vi "LaserStatus.vi"() -> (0 "h1-transmission":dbl format="%.2f", 1 "rep-rate":dbl format="%.2f", 2 "hu-error-code":i32, 3 "laser-error-code":i32, 4 "h1-zero-transmission-offset":i32, 5 "HU-Temp-Ready?":bool, 6 "LD1-set-current":dbl format="%.2f", 7 "LaserOn?":bool)   [LabVIEW 2020]
uses:
  <vilib>/JDP Science/JSONtext/String Subset.vi
  <vilib>/JDP Science/JSONtext/Parsing/Parse Full Path or Item Name.vi
  <vilib>/JDP Science/JSONtext/Next JSON Value.vi
  <vilib>/JDP Science/JSONtext/support/Error Cluster From Code.vi
  <vilib>/JDP Science/JSONtext/Offset/Find Item Locations by Path.vi
  <vilib>/httpClient/LabVIEWHTTPClient.lvlib
  <vilib>/JDP Science/JSONtext/JSONtext.lvlib
panel:
  out "body":string
  out "headers":string
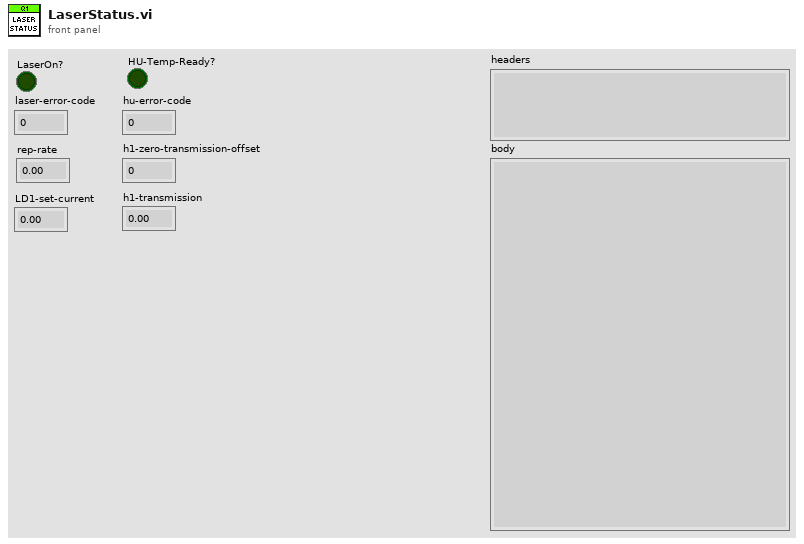
[diagram p1: front panel]
types:
  T1 = typedef "LabVIEWHTTPClient.lvlib/ClientHandle.ctl" = refnum<k1>
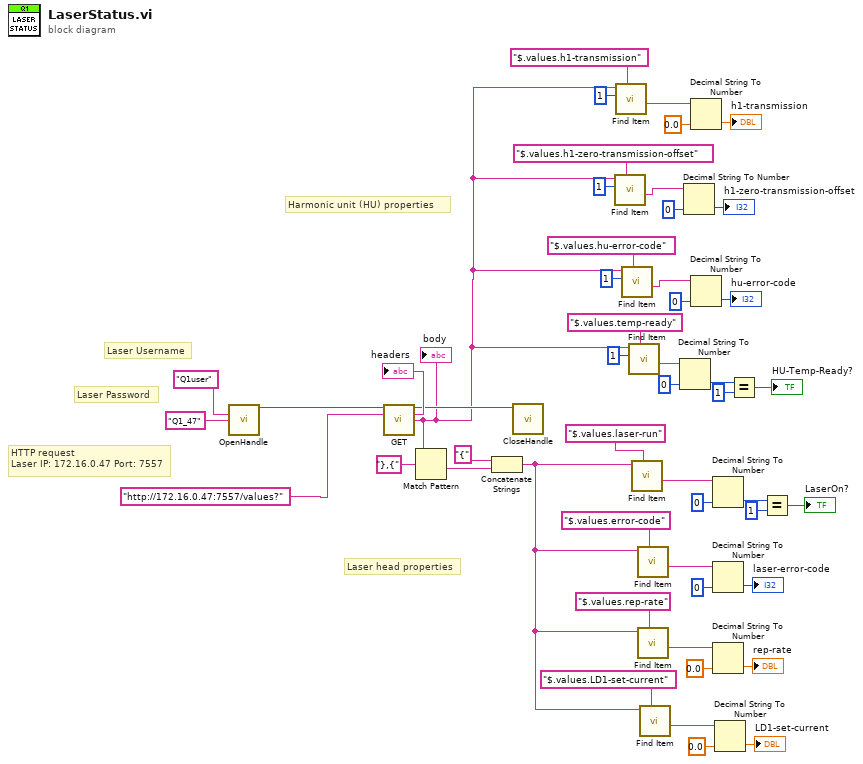
[diagram p0: block diagram]
diagram:
  # "Harmonic unit (HU) properties"
  # "Laser head properties"
  # "HTTP request\nLaser IP: 172.16.0.47 Port: 7557"
  # "Laser Password"
  # "Laser Username"
  n1 = call <vilib>:"OpenHandle.vi"("username"="Q1user", "password"="Q1_47") -> ("client handle out"=w50:T1)  [unwired: 12 in, 1 out]
  n2 = call <vilib>:"GET.vi"("client handle"=w50, "url"="http://172.16.0.47:7557/values?") -> ("client handle out"=w47:T1, "headers"=→"headers":string, "body"=w3:string)  [unwired: 10 in, 1 out]
  "body" <- w3
  n3 = Match Pattern(string=w3, regular expression="},{") -> (after substring=w42:string)  [unwired: 1 in, 3 out]
  n4 = Concatenate Strings("{" ("string"), w42) -> (w24:string)
  n5 = call <vilib>:"CloseHandle.vi"("client handle"=w47) -> ()  [unwired: 14 in, 1 out]
  n6 = call <vilib>:"Find Item.vi"("$Path or Item Name"="$.values.h1-zero-transmission-offset", "Offset"=1, "JSON"=w3) -> ("<JSON>"=w7:string)  [unwired: 5 in, 3 out]
  n7 = call <vilib>:"Find Item.vi"("$Path or Item Name"="$.values.h1-transmission", "Offset"=1, "JSON"=w3) -> ("<JSON>"=w5:string)  [unwired: 5 in, 3 out]
  n8 = call <vilib>:"Find Item.vi"("$Path or Item Name"="$.values.hu-error-code", "Offset"=1, "JSON"=w3) -> ("<JSON>"=w12:string)  [unwired: 5 in, 3 out]
  n9 = call <vilib>:"Find Item.vi"("$Path or Item Name"="$.values.temp-ready", "Offset"=1, "JSON"=w3) -> ("<JSON>"=w17:string)  [unwired: 5 in, 3 out]
  n10 = call <vilib>:"Find Item.vi"("$Path or Item Name"="$.values.laser-run", "JSON"=w24) -> ("<JSON>"=w41:string)  [unwired: 6 in, 3 out]
  n11 = call <vilib>:"Find Item.vi"("$Path or Item Name"="$.values.error-code", "JSON"=w24) -> ("<JSON>"=w34:string)  [unwired: 6 in, 3 out]
  n12 = call <vilib>:"Find Item.vi"("$Path or Item Name"="$.values.rep-rate", "JSON"=w24) -> ("<JSON>"=w30:string)  [unwired: 6 in, 3 out]
  n13 = call <vilib>:"Find Item.vi"("$Path or Item Name"="$.values.LD1-set-current", "JSON"=w24) -> ("<JSON>"=w27:string)  [unwired: 6 in, 3 out]
  n14 = Decimal String To Number(string=w17, default (0L)=0 ("default (0 I32)")) -> (number=w20:i32)  [unwired: 1 in, 1 out]
  n15 = Decimal String To Number(string=w7, default (0L)=0 ("default (0 I32)")) -> (number=→"h1-zero-transmission-offset":i32)  [unwired: 1 in, 1 out]
  n16 = Decimal String To Number(string=w5, default (0L)=0.0 ("default (0 I32)")) -> (number=→"h1-transmission":dbl)  [unwired: 1 in, 1 out]
  n17 = Decimal String To Number(string=w12, default (0L)=0 ("default (0 I32)")) -> (number=→"hu-error-code":i32)  [unwired: 1 in, 1 out]
  n18 = Decimal String To Number(string=w41, default (0L)=0 ("default (0 I32)")) -> (number=w39:i32)  [unwired: 1 in, 1 out]
  n19 = Decimal String To Number(string=w34, default (0L)=0 ("default (0 I32)")) -> (number=→"laser-error-code":i32)  [unwired: 1 in, 1 out]
  n20 = Decimal String To Number(string=w30, default (0L)=0.0 ("default (0 I32)")) -> (number=→"rep-rate":dbl)  [unwired: 1 in, 1 out]
  n21 = Decimal String To Number(string=w27, default (0L)=0.0 ("default (0 I32)")) -> (number=→"LD1-set-current":dbl)  [unwired: 1 in, 1 out]
  n22 = Equal?(x=w20, y=1) -> (x = y?=→"HU-Temp-Ready?":bool)
  n23 = Equal?(x=w39, y=1) -> (x = y?=→"LaserOn?":bool)
